vi "Auto_timed_cube in+drive.vi"(2 "Cube In Speed":dbl, 3 "Cube In Time":dbl, 4 "Drive Speed":dbl, 5 "RobotDriveDevRef in":T1) -> (1 "RobotDriveDevRef out":T1)   [LabVIEW 2017]
uses:
  <vilib>/Rock Robotics/WPI/RobotDrive/WPI_RobotDriveDevRef.ctl
  <vilib>/Rock Robotics/WPI/MotorControl/WPI_MotorControlDeviceRef.ctl
  <vilib>/Rock Robotics/WPI/MotorControl/WPI_MotorControlType.ctl
  <vilib>/Rock Robotics/SystemInterfaces/DIO/FPGA_DIOPWMChannel.ctl
  <vilib>/Rock Robotics/WPI/PWM/WPI_PWMDeadband.ctl
  <vilib>/Rock Robotics/SystemInterfaces/DIO/FPGA_DIOChannel.ctl
  <vilib>/Rock Robotics/WPI/RobotDrive/WPI_RobotDriveArcadeDrive_Standard(NoSaturation).vi
panel:
  in  "Axes[3]":dbl
  in  "Axes[2]":dbl
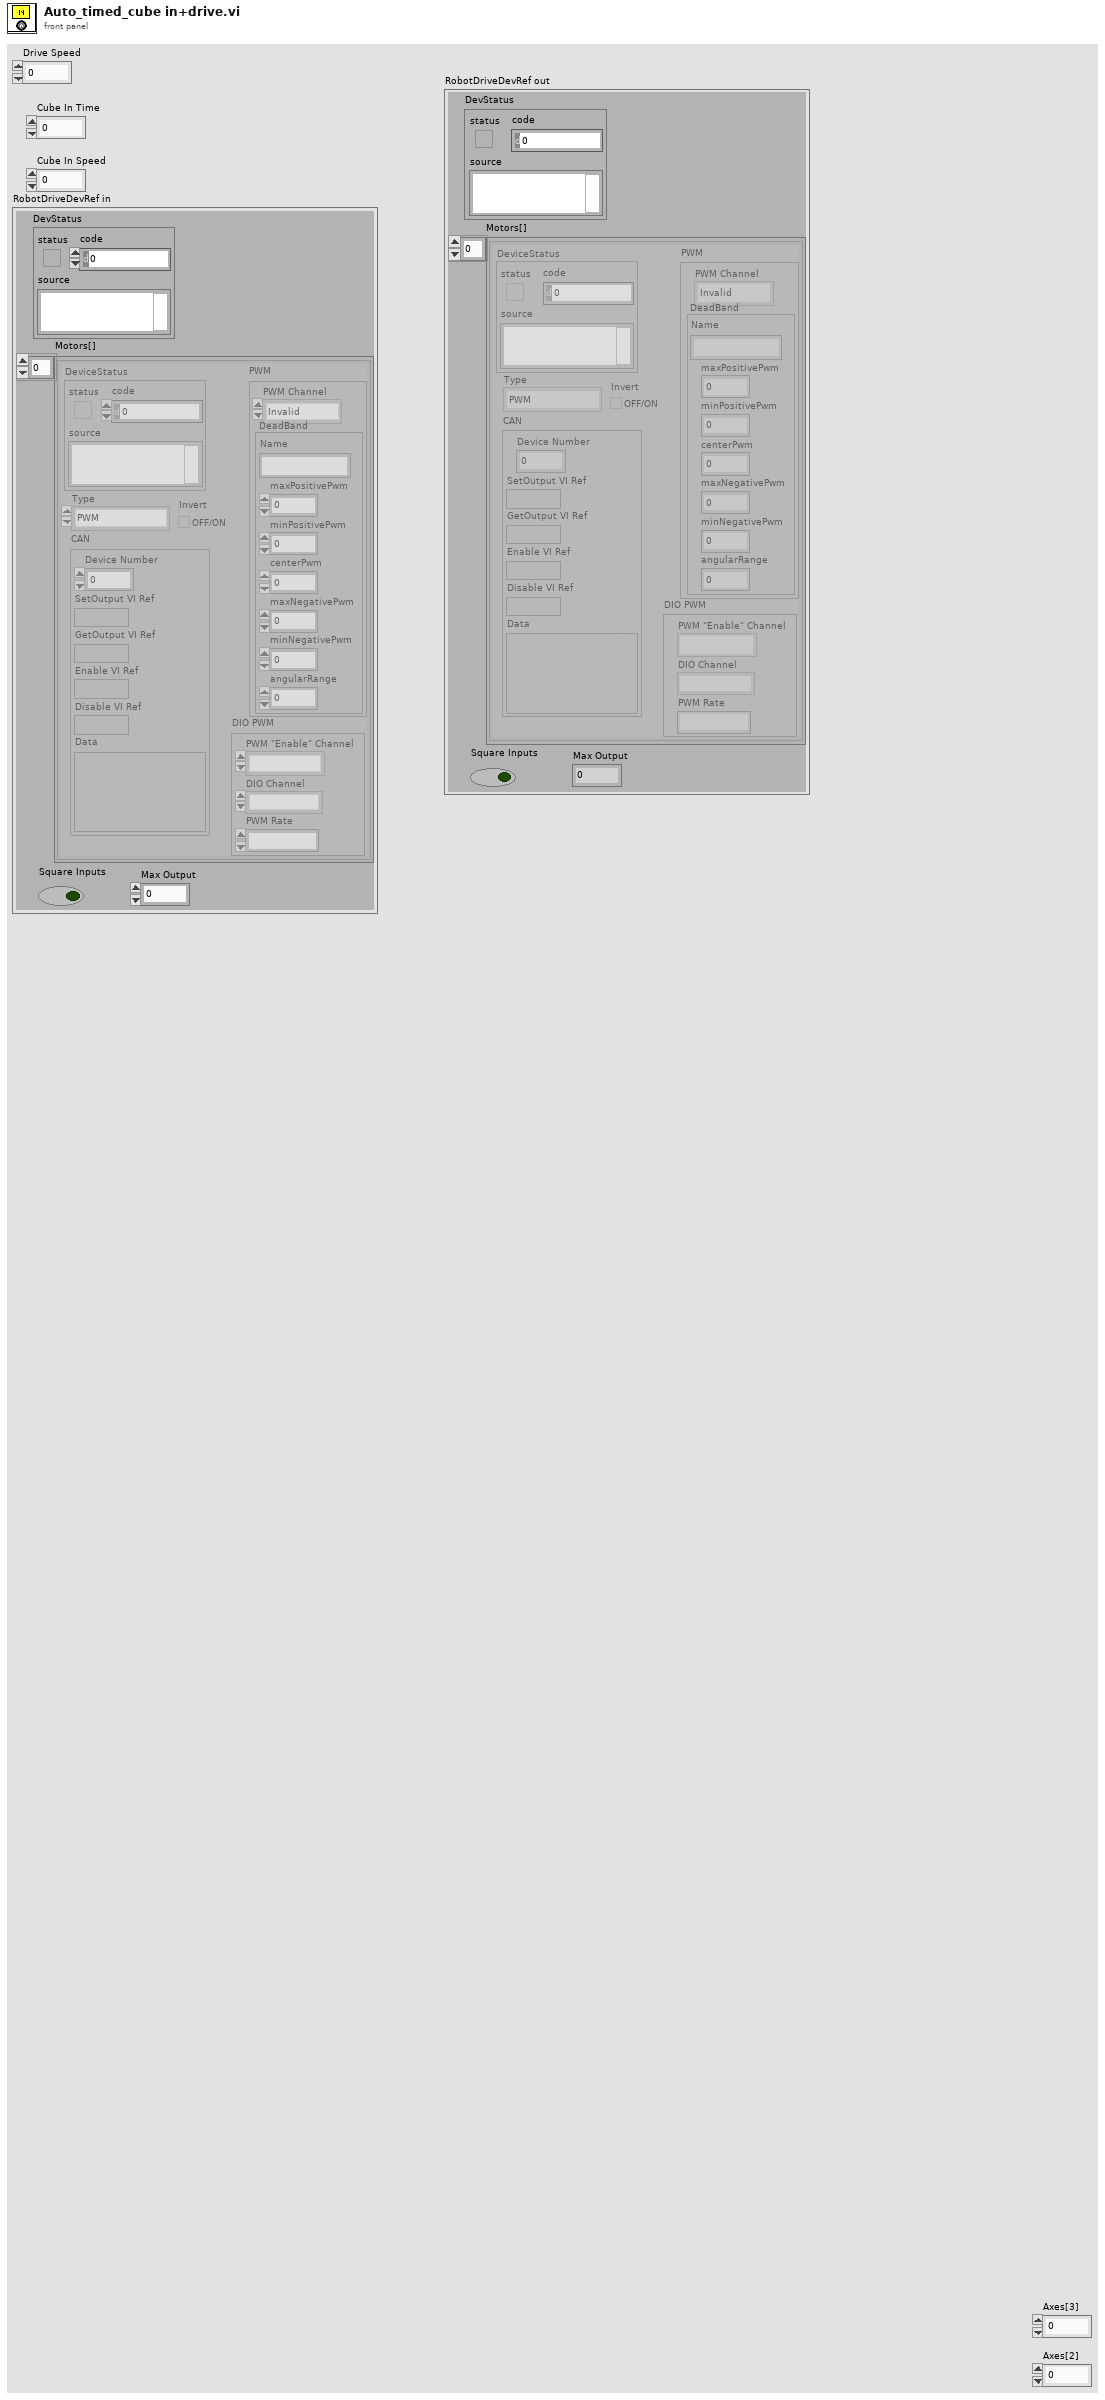
[diagram p1: front panel]
types:
  T1 = typedef "WPI_RobotDriveDevRef.ctl" = cluster{"DevStatus":errorcluster, "Motors[]":T2[], "Square Inputs":bool, "Max Output":dbl}
  T2 = typedef "WPI_MotorControlDeviceRef.ctl" = cluster{"DeviceStatus":errorcluster, "Type":T3, "PWM":cluster{"PWM Channel":T4, "DeadBand":T5}, "CAN":cluster{"Device Number":u8, "SetOutput VI Ref":variant, "GetOutput VI Ref":variant, "Enable VI Ref":variant, "Disable VI Ref":variant, "Data":variant}, "Invert":bool, "DIO PWM":cluster{"PWM \"Enable\" Channel":T4, "DIOChannel":T6, "PWM Rate":dbl}}
  T3 = typedef "WPI_MotorControlType.ctl" = enum16{"PWM", "CAN", "DIO PWM"}
  T4 = typedef "FPGA_DIOPWMChannel.ctl" = enum8{"PWM 0", "PWM 1", "PWM 2", "PWM 3", "PWM 4", "PWM 5", "PWM 6", "PWM 7", "PWM 8", "PWM 9", "PWM MXP 0", "PWM MXP 1", "PWM MXP 2", "PWM MXP 3", "PWM MXP 4", "PWM MXP 5", "PWM MXP 6", "PWM MXP 7", "PWM MXP 8", "PWM MXP 9", "Invalid"}
  T5 = typedef "WPI_PWMDeadband.ctl" = cluster{"Name":string, "maxPositivePwm":i32, "minPositivePwm":i32, "centerPwm":i32, "maxNegativePwm":i32, "minNegativePwm":i32, "angularRange":u16}
  T6 = typedef "FPGA_DIOChannel.ctl" = enum8{"DIO 0", "DIO 1", "DIO 2", "DIO 3", "DIO 4", "DIO 5", "DIO 6", "DIO 7", "DIO 8", "DIO 9", "DIO MXP 0", "DIO MXP 1", "DIO MXP 2", "DIO MXP 3", "DIO MXP 4", "DIO MXP 5", "DIO MXP 6", "DIO MXP 7", "DIO MXP 8", "DIO MXP 9", "DIO MXP 10", "DIO MXP 11", "DIO MXP 12", "DIO MXP 13", "DIO MXP 14", "DIO MXP 15", "SPI Port CS1", "SPI Port CS2", "SPI Port CS3", "SPI Port MISO", "SPI Port MOSI", "Invalid"}
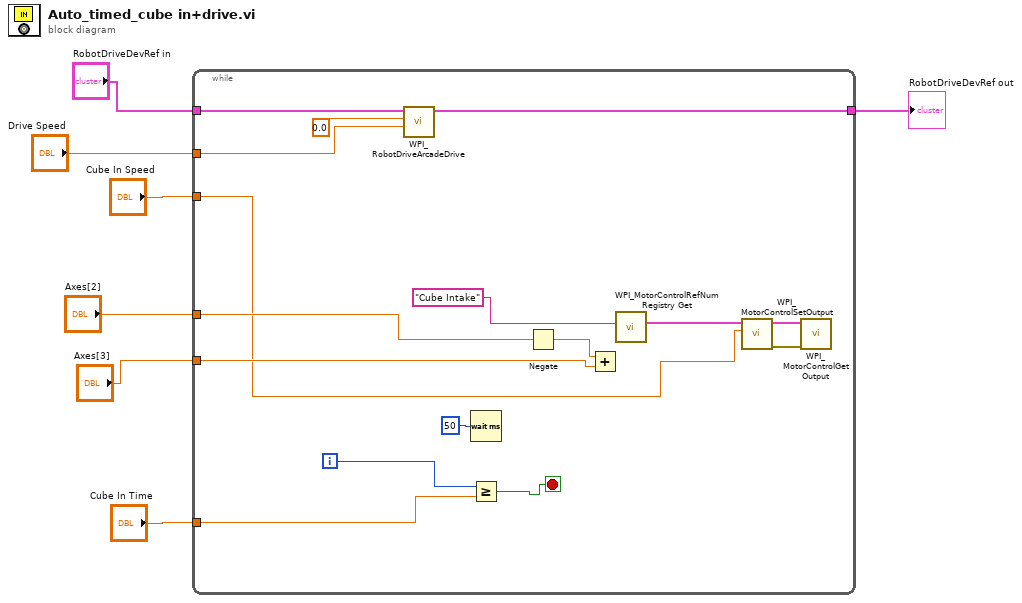
[diagram p0: block diagram]
diagram:
  n1 = while {
    tunnel: "Cube In Speed" -> [w9]
    tunnel: "Cube In Time" -> [w20]
    tunnel: "RobotDriveDevRef in" -> [w18]
    tunnel: [w17] -> w4
    tunnel: "Axes[3]" -> [w11]
    tunnel: "Axes[2]" -> [w10]
    tunnel: "Drive Speed" -> [w8]
    i -> [w21]
    stop <- w23 stop-if-true
    n2 = call-poly <vilib>:"WPI_RobotDriveArcadeDrive.vi"("Y axis value"=w8, "X axis value"=0.0, "RobotDriveDevRef"=w18) -> ("RobotDriveDevRef"=w17:T1)  [unwired: 1 in, 7 out]
    n3 = Wait (ms)(milliseconds to wait=50) -> ()  [unwired: 1 out]
    n4 = Greater Or Equal?(x=w21, y=w20) -> (x >= y?=w23:bool)
    n5 = Negate(x=w10) -> (-x=w13:dbl)
    n6 = Add(x=w13, y=w11) -> ()  [unwired: 1 out]
    n7 = call <vilib>:"WPI_MotorControlRefNum Registry Get.vi"("refnum name"="Cube Intake") -> ("MotorControlDevRef"=w15:T2)  [unwired: 9 in, 1 out]
    n8 = call <vilib>:"WPI_MotorControlSetOutput.vi"("Output"=w9, "MotorControlDevRef"=w15) -> ("error out"=w14:errorcluster, "MotorControlDevRef"=w16:T2)  [unwired: 7 in, 1 out]
    n9 = call <vilib>:"WPI_MotorControlGetOutput.vi"("error in (no error)"=w14, "MotorControlDevRef"=w16) -> ()  [unwired: 7 in, 3 out]
  }
  "RobotDriveDevRef out" <- w4
